vi "rtin_controlAQuadBInResolution.vi"(7 "Set":bool, 8 "error in":errorcluster, 9 "amplitude [V] in":i32, 10 "axis in":u8, 11 "connection ID":refnum<k5>) -> (0 "error out":errorcluster, 1 "amplitude [V] out":i32, 2 "axis out":i32, 3 "connection ID":refnum<k5>)   [LabVIEW 2016, in "AMC_VIs.lvlib"]
doc: "This function retrieves or sets the AQuadB input resolution for setpoint parameter."
uses:
  AMC_VIs.lvlib
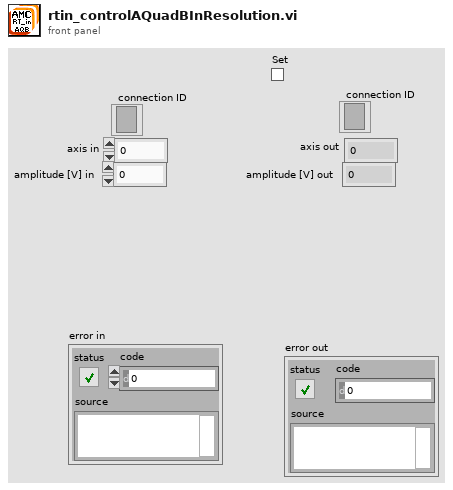
[diagram p1: front panel]
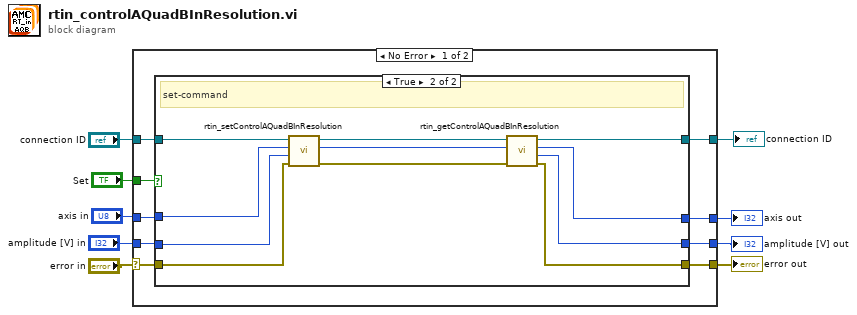
[diagram p0: block diagram]
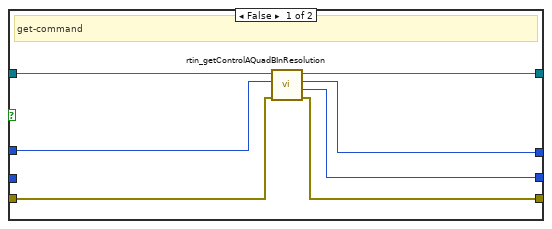
[diagram p2: hidden frame]
diagram:
  n1 = case shown="No Error" "error in" {
    selector: "error in" -> [w14 w40]
    tunnel: "axis in" -> [w18 w37]
    tunnel: [w11 w40] -> w8
    tunnel: "amplitude [V] in" -> [w16 w38]
    tunnel: [w13 w38] -> w3
    tunnel: "Set" -> [w15 _]
    tunnel: [w12 w39] -> w6
    tunnel: "connection ID" -> [w17 w39]
    tunnel: [w10 w37] -> w1
    frame No Error {
      n2 = case shown="True" w15 {
        tunnel: w17 -> [w20 w33]
        tunnel: w18 -> [w19 w30]
        tunnel: w16 -> [_ w27]
        tunnel: w14 -> [w21 w31]
        tunnel: [w22 w26] -> w13
        tunnel: [w24 w32] -> w12
        tunnel: [w25 w29] -> w11
        tunnel: [w23 w28] -> w10
        frame False {
          # "get-command"
          n3 = call "rtin_getControlAQuadBInResolution.vi"("error in"=w21, "axis"=w19, "connection ID"=w20) -> ("error out"=w25:errorcluster, "resolution"=w22:i32, "axis_out"=w23:i32, "connection ID"=w24:refnum<k5>)  [unwired: 5 in]
        }
        frame True {
          # "set-command"
          n4 = call "rtin_setControlAQuadBInResolution.vi"("error in"=w31, "resolution"=w27, "axis"=w30, "connection ID"=w33) -> ("error out"=w34:errorcluster, "axis_out"=w36:i32, "connection ID"=w35:refnum<k5>)  [unwired: 5 in]
          n5 = call "rtin_getControlAQuadBInResolution.vi"("error in"=w34, "axis"=w36, "connection ID"=w35) -> ("error out"=w29:errorcluster, "resolution"=w26:i32, "axis_out"=w28:i32, "connection ID"=w32:refnum<k5>)  [unwired: 5 in]
        }
      }
    }
    frame Error {
    }
  }
  "error out" <- w8
  "axis out" <- w1
  "amplitude [V] out" <- w3
  "connection ID" <- w6
